vi "Map - Set.vi"(8 "error in (no error)":errorcluster, 9 "Value":variant, 10 "Key":string, 11 "Map In":variant) -> (0 "error out":errorcluster, 2 "Replaced?":bool, 3 "Map Out":variant)   [LabVIEW 2024]
doc: "Sets a node in <b>Map</b>."
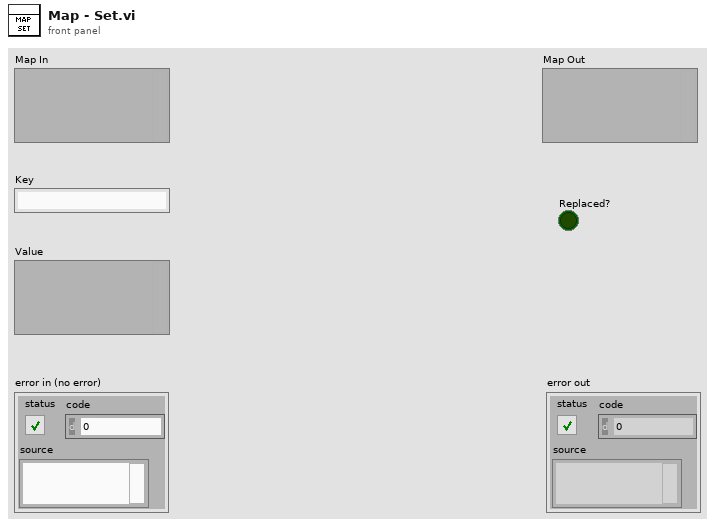
[diagram p1: front panel]
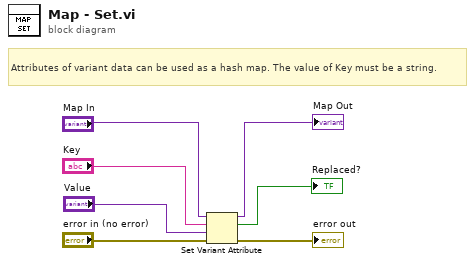
[diagram p0: block diagram]
diagram:
  # "Attributes of variant data can be used as a hash map. The value of Key must be a string."
  n1 = Set Variant Attribute(Variant="Map In", name="Key", value="Value", error in="error in (no error)") -> (Variant out=→"Map Out":variant, replaced=→"Replaced?":bool, error out=→"error out":errorcluster)
